vi "SPINE (SubVI).vi"(0 "Input Valid?":bool, 1 "Skip SPLINE?":bool, 2 "HT Location":u64[](array[numeric])=[0, 0, 0, 0, 0, 0, 0, 0, 0, 0, 0, 0, 0, 0, 0, 0], 3 "V1 (ID)":u16, 4 "V2 (ID)":u16, 5 "N Points":u16, 6 "N Spline Points":fxp<+,8,8>=31.0) -> (13 "Ready for Input?":bool)   [LabVIEW 2015]
uses:
  Controls (FPGA)/Fixed Point Contour.ctl
  <vilib>/rvi/FXPMathLib/FxpDiv/subVIs/nifxpmath_Div_SimConfig.ctl
  <vilib>/rvi/Emulation/niFpgaProcessEmulError.vi
  <vilib>/rvi/DataTransferAndStorage/Container/Common/niFpgaContainerGetUniqueNameForEmu.vi
  <vilib>/rvi/DataTransferAndStorage/Container/Common/niFpgaContainerSetEmuInfo.vi
  <vilib>/rvi/eio/common/nirviEmuReportErrorAndStop.vi
  <vilib>/rvi/Emulation/niFpgaEmulationIsFPGAContextNoSignature.vi
  <vilib>/rvi/Memory/Memory_Emulation/niFpgaMemoryEmulationCacheClearOnFirstRun.vi
  <vilib>/rvi/Memory/Memory_Emulation/nirvimemoryEmulationManagerCache_MakeExclusive.vi
  <vilib>/rvi/Memory/Memory_Emulation/niFpgaMemoryEmulationValidateCache.vi
  <vilib>/rvi/Memory/Memory_Emulation/nirvimemoryEmulationManagerCache_InsertValue.vi
  <vilib>/Utility/error.llb/Clear Errors.vi
  <vilib>/rvi/Memory/Memory_Emulation/nirvimemoryEmulationManagerCache_ReleaseExclusive.vi
  <vilib>/rvi/Memory/Memory_Emulation/nirvimemoryEmulationManagerCache_GetValue.vi
  <vilib>/rvi/Memory/Memory_Emulation/nirvimemoryEmulationManagerCache_SetValue.vi
  <vilib>/rvi/Emulation/niFpgaSctlEmulationGetInTimedLoop.vi
  <vilib>/rvi/interface/RandomDataEmulation/niFpgaRandomDataHandleErrors.vi
  <vilib>/rvi/Memory/Memory_Emulation/nirvimemoryFastEmulation.vi
  <vilib>/rvi/Memory/Memory_Emulation/nirvimemoryEmulation.vi
  <vilib>/rvi/errors/nirviReportUnexpectedCaseInternalError (U32).vi
  <vilib>/rvi/FXPMathLib/FxpDiv/simVIs/DllFxpDivTemp_sub.vi
  <vilib>/rvi/LocalResourceManager/LocalResourceManager.xnode
  <vilib>/rvi/DataTransferAndStorage/Container/XNode/niFpgaContainer.xnode
  <vilib>/rvi/DataTransferAndStorage/Register/Emulation/niFpgaRegisterEmulation.vi
  <vilib>/rvi/interface/RandomDataEmulation/nirviRandomDataFpgaReadWriteTemplate.vi
  <vilib>/rvi/FXPMathLib/FxpDiv/XNode/nifxpmath_Div.xnode
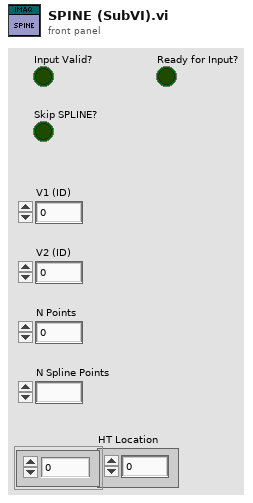
[diagram p1: front panel]
types:
  T1 = typedef "Fixed Point Contour.ctl" = enum16{"Wait", "Read Point 1", "Read Point 2"}
  T2 = cluster{"Int1":fxp<+/-,24,16>, "Int2":fxp<+/-,24,16>}
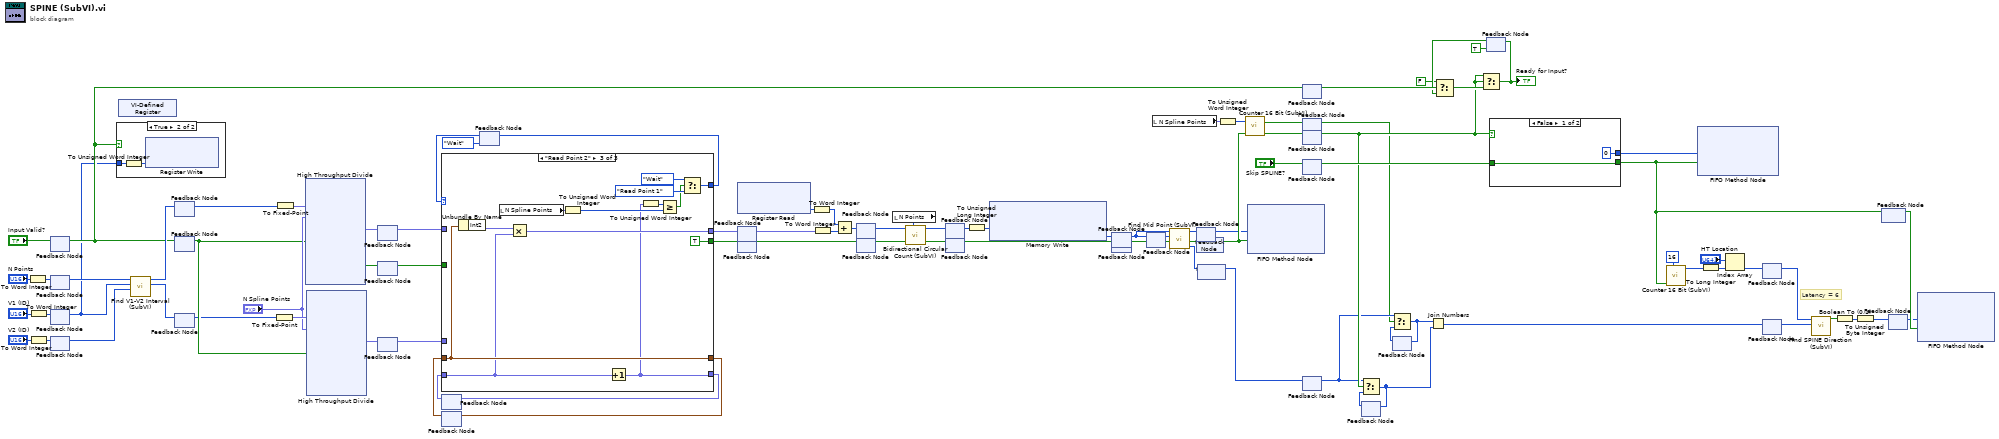
[diagram p0: block diagram]
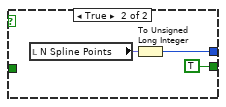
[diagram p3: hidden frame]
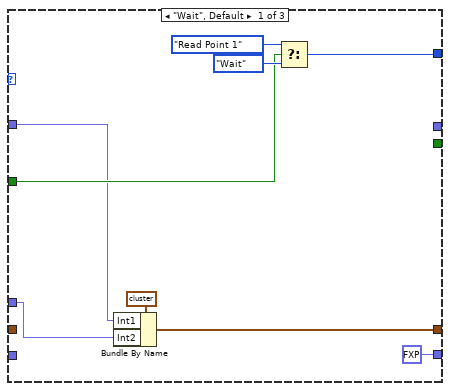
[diagram p4: hidden frame]
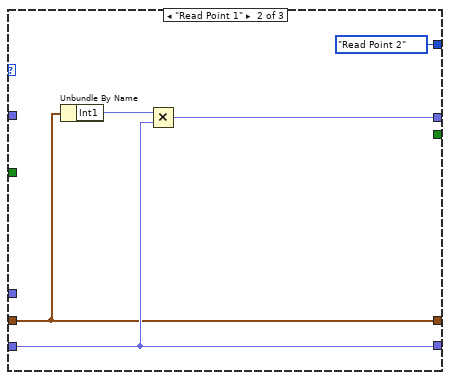
[diagram p5: hidden frame]
diagram:
  # "Latency = 6"
  n1 = To Word Integer(number="N Points") -> (16bit integer=w34:i16)
  n2 = To Word Integer(number="V1 (ID)") -> (16bit integer=w33:i16)
  n3 = To Word Integer(number="V2 (ID)") -> (16bit integer=w32:i16)
  n4 = feedback-in #1("Input Valid?") -> ()
  n5 = feedback #1() -> (w31:bool)  [unwired: 1 in]
  n6 = feedback-in #2(w34) -> ()
  n7 = feedback #2() -> (w86:i16)  [unwired: 1 in]
  n8 = feedback-in #3(w33) -> ()
  n9 = feedback #3() -> (w26:i16)  [unwired: 1 in]
  n10 = feedback-in #4(w32) -> ()
  n11 = feedback #4() -> (w27:i16)  [unwired: 1 in]
  n12 = case shown="True" w31 {
    tunnel: w26 -> [_ w92]
    frame False {
    }
    frame True {
      n13 = To Unsigned Word Integer(number=w92) -> (unsigned 16bit integer=w91:u16)
      n14 = xnode ("Register Write")("Data"=w91) -> ()  [unwired: 1 in, 1 out]
    }
  }
  n15 = xnode "VI-Defined Register"() -> ()  [unwired: 1 out]
  n16 = call "Find V1-V2 Interval (SubVI).vi"("V2"=w27, "V1"=w26, "N Points"=w86) -> ("V2-V1"=w83:i16, "V1-V2"=w85:i16)  [unwired: 7 in]
  n17 = feedback-in #5(w85) -> ()
  n18 = feedback #5() -> (w29:i16)  [unwired: 1 in]
  n19 = feedback-in #6(w31) -> ()
  n20 = feedback #6() -> (w30:bool)  [unwired: 1 in]
  n21 = feedback-in #7(w83) -> ()
  n22 = feedback #7() -> (w28:i16)  [unwired: 1 in]
  n23 = To Fixed-Point(number=w28) -> (fixed-point=w82:fxp<+/-,16,16>)  [unwired: 1 in]
  n24 = To Fixed-Point(number=w29) -> (fixed-point=w84:fxp<+/-,16,16>)  [unwired: 1 in]
  n25 = xnode "High Throughput Divide"("x"=w84, "y"="N Spline Points", "input valid"=w30) -> ("x/y"=w79:fxp<+/-,24,16>, "output valid"=w70:bool)  [unwired: 1 in, 1 out]
  n26 = xnode "High Throughput Divide"("x"=w82, "y"="N Spline Points", "input valid"=w30) -> ("x/y"=w80:fxp<+/-,24,16>)  [unwired: 1 in, 2 out]
  n27 = feedback-in #8(w79) -> ()
  n28 = feedback #8() -> (w75:fxp<+/-,24,16>)  [unwired: 1 in]
  n29 = feedback-in #9(w70) -> ()
  n30 = feedback #9() -> (w73:bool)  [unwired: 1 in]
  n31 = feedback-in #10(w80) -> ()
  n32 = feedback #10() -> (w74:fxp<+/-,24,16>)  [unwired: 1 in]
  n33 = feedback #11() -> (w68:fxp<+,16,16>)  [unwired: 1 in]
  n34 = feedback #12() -> (w71:T2)  [unwired: 1 in]
  n35 = feedback #13(Fixed_Point_Contour."Wait") -> (w77:T1)
  n36 = case shown="\"Read Point 2\"" w77 {
    tunnel: w74 -> [w95 _ _]
    tunnel: w75 -> [w96 _ _]
    tunnel: [w100 Fixed_Point_Contour."Read Point 2" w117] -> w78
    tunnel: w73 -> [w99 _ _]
    tunnel: [w94 w104 w112] -> w72
    tunnel: w71 -> [_ w104 w112]
    tunnel: [fxp<+,16,16> 0.0 ("N Points") w105 w109] -> w69
    tunnel: w68 -> [_ w105 w108]
    tunnel: [_ w102 w111] -> w50
    tunnel: [_ _ TRUE] -> w65
    frame "Wait", Default {
      n37 = Bundle By Name(cluster=T2 {"Int1"=0.0, "Int2"=0.0}, "Int1"=w96, "Int2"=w95) -> (w94:T2)
      n38 = Select(t=Fixed_Point_Contour."Read Point 1", s=w99, f=Fixed_Point_Contour."Wait") -> (s? t:f=w100:T1)
    }
    frame "Read Point 1" {
      n39 = Unbundle By Name(w104) -> ("Int1"=w103:fxp<+/-,24,16>)
      n40 = Multiply(x=w103, y=w105) -> (x*y=w102:fxp<+/-,40,32>)
    }
    frame "Read Point 2" {
      n41 = Unbundle By Name(w112) -> ("Int2"=w113:fxp<+/-,24,16>)
      n42 = local read "N Spline Points"() -> (w116:fxp<+,8,8>)
      n43 = Multiply(x=w113, y=w108) -> (x*y=w111:fxp<+/-,40,32>)
      n44 = To Unsigned Word Integer(number=w116) -> (unsigned 16bit integer=w110:u16)
      n45 = Increment(x=w108) -> (x+1=w109:fxp<+,16,16>)
      n46 = To Unsigned Word Integer(number=w109) -> (unsigned 16bit integer=w107:u16)
      n47 = Greater Or Equal?(x=w107, y=w110) -> (x >= y?=w114:bool)
      n48 = Select(t=Fixed_Point_Contour."Wait", s=w114, f=Fixed_Point_Contour."Read Point 1") -> (s? t:f=w117:T1)
    }
  }
  n49 = feedback-in #11(w69) -> ()
  n50 = feedback-in #12(w72) -> ()
  n51 = feedback-in #13(w78) -> ()
  n52 = xnode ("Register Read")() -> ("Data"=w51:u16)  [unwired: 1 in, 1 out]
  n53 = feedback-in #14(w50) -> ()
  n54 = feedback #14() -> (w47:fxp<+/-,40,32>)  [unwired: 1 in]
  n55 = feedback-in #15(w65) -> ()
  n56 = feedback #15() -> (w46:bool)  [unwired: 1 in]
  n57 = To Word Integer(number=w51) -> (16bit integer=w52:i16)
  n58 = To Word Integer(number=w47) -> (16bit integer=w48:i16)
  n59 = Add(x=w52, y=w48) -> (x+y=w49:i16)
  n60 = feedback-in #16(w49) -> ()
  n61 = feedback #16() -> (w56:i16)  [unwired: 1 in]
  n62 = feedback-in #17(w46) -> ()
  n63 = feedback #17() -> (w55:bool)  [unwired: 1 in]
  n64 = local read "N Points"() -> (w59:u16)
  n65 = call "Bidirectional Circular Count (SubVI).vi"("Max. Count"=w59, "Count In"=w56) -> ("Count Out"=w58:i16)  [unwired: 9 in]
  n66 = feedback-in #18(w58) -> ()
  n67 = feedback #18() -> (w54:i16)  [unwired: 1 in]
  n68 = feedback-in #19(w55) -> ()
  n69 = feedback #19() -> (w53:bool)  [unwired: 1 in]
  n70 = To Unsigned Long Integer(number=w54) -> (unsigned 32bit integer=w57:u32)
  n71 = xnode ("Memory Write")("Address"=w57) -> ("Data"=w67:u32)  [unwired: 1 in, 1 out]
  n72 = feedback #20() -> (w62:u32)  [unwired: 1 in]
  n73 = feedback-in #20(w67) -> ()
  n74 = feedback-in #21(w53) -> ()
  n75 = feedback #21() -> (w64:bool)  [unwired: 1 in]
  n76 = feedback #22() -> (w63:u32)  [unwired: 1 in]
  n77 = feedback-in #22(w62) -> ()
  n78 = local read "N Spline Points"() -> (w61:fxp<+,8,8>)
  n79 = call "Find Mid Point (SubVI).vi"("Point 2"=w63, "Point 1"=w62) -> ("Mid Point (Int)"=w4:u32, "Mid Point"=w66:u32)  [unwired: 8 in]
  n80 = feedback-in #23(w66) -> ()
  n81 = feedback #23() -> (w3:u32)  [unwired: 1 in]
  n82 = feedback-in #24(w64) -> ()
  n83 = feedback #24() -> (w37:bool)  [unwired: 1 in]
  n84 = feedback #25() -> (w2:u32)  [unwired: 1 in]
  n85 = feedback-in #25(w4) -> ()
  n86 = To Unsigned Word Integer(number=w61) -> (unsigned 16bit integer=w60:u16)
  n87 = call "Counter 16 Bit (SubVI).vi"("Max. Count"=w60, "Enable"=w37) -> ("Count Begin?"=w15:bool, "Count End?"=w36:bool)  [unwired: 11 in, 1 out]
  n88 = xnode ("FIFO Method Node")("Element"=w3, "Input Valid"=w37) -> ()  [unwired: 1 in, 2 out]
  n89 = feedback #26() -> (w45:bool)  [unwired: 1 in]
  n90 = feedback-in #26(w31) -> ()
  n91 = feedback-in #27(w15) -> ()
  n92 = feedback #27() -> (w14:bool)  [unwired: 1 in]
  n93 = feedback-in #28(w36) -> ()
  n94 = feedback #28() -> (w18:bool)  [unwired: 1 in]
  n95 = feedback #29() -> (w35:bool)  [unwired: 1 in]
  n96 = feedback-in #29("Skip SPLINE?") -> ()
  n97 = feedback-in #30(w2) -> ()
  n98 = feedback #30() -> (w16:u32)  [unwired: 1 in]
  n99 = feedback #31() -> (w19:u32)  [unwired: 1 in]
  n100 = Select(t=w16, s=w18, f=w19) -> (s? t:f=w13:u32)
  n101 = feedback-in #31(w13) -> ()
  n102 = feedback #32() -> (w17:u32)  [unwired: 1 in]
  n103 = Select(t=w16, s=w14, f=w17) -> (s? t:f=w1:u32)
  n104 = feedback-in #32(w1) -> ()
  n105 = Join Numbers(hi=w1, lo=w13) -> ((hi.lo)=w12:u64)
  n106 = feedback #33(TRUE ("t")) -> (w43:bool)
  n107 = Select(t=FALSE, s=w45, f=w43) -> (s? t:f=w44:bool)
  n108 = Select(t=w18, s=w18, f=w44) -> (s? t:f=w42:bool)
  "Ready for Input?" <- w42
  n109 = feedback-in #33(w42) -> ()
  n110 = case shown="False" w18 {
    tunnel: [u32 0 w123] -> w38
    tunnel: [w120 TRUE ("t")] -> w9
    tunnel: w35 -> [w120 _]
    frame False {
    }
    frame True {
      n111 = local read "N Spline Points"() -> (w124:fxp<+,8,8>)
      n112 = To Unsigned Long Integer(number=w124) -> (unsigned 32bit integer=w123:u32)
    }
  }
  n113 = call "Counter 16 Bit (SubVI).vi"("Max. Count"=u16 16, "Enable"=w9) -> ("Count"=w24:u16)  [unwired: 11 in, 2 out]
  n114 = xnode ("FIFO Method Node")("Element"=w38, "Input Valid"=w9) -> ()  [unwired: 1 in, 2 out]
  n115 = To Long Integer(number=w24) -> (32bit integer=w22:i32)
  n116 = Index Array(array="HT Location", index=w22) -> (element=w21:u64)
  n117 = feedback #34() -> (w11:u64)  [unwired: 1 in]
  n118 = feedback-in #34(w21) -> ()
  n119 = feedback #35() -> (w20:u64)  [unwired: 1 in]
  n120 = feedback-in #35(w12) -> ()
  n121 = call "Find SPINE Direction (SubVI).vi"("Point 2"=w20, "Point 1"=w11) -> ("Reverse?"=w10:bool)  [unwired: 9 in]
  n122 = Boolean To (0,1)(Boolean=w10) -> (0, 1=w7:i16)
  n123 = To Unsigned Byte Integer(number=w7) -> (unsigned 8bit integer=w6:u8)
  n124 = feedback #36() -> (w8:bool)  [unwired: 1 in]
  n125 = feedback-in #36(w9) -> ()
  n126 = feedback-in #37(w6) -> ()
  n127 = feedback #37() -> (w5:u8)  [unwired: 1 in]
  n128 = xnode ("FIFO Method Node")("Element"=w5, "Input Valid"=w8) -> ()  [unwired: 1 in, 2 out]
